vi "SFP_SwitchDMM.vi"(11 "DMM Instrument":refnum<class "DMM Instrument.lvclass">) -> ()   [LabVIEW 2025]
doc: "Copyright 2017 National Instruments Corporation\n\nLicensed under the Apache License, Version 2.0 (the \"License\"); you may not use this file except in compliance with the License. You may obtain a copy of the License at http://www.apache.org/licenses/LICENSE-2.0\nUnless required by applicable law or agreed to in writing, software distributed under the License is distributed on an \"AS IS\" BASIS, WITHOUT WARRANTIES OR CONDITIONS OF ANY KIND, either express or implied. See the License for the specific language governing permissions and limitations under the License."
uses:
  DMM Instrument.lvclass/DMM Instrument.ctl
  DMM Instrument.lvclass
  C:/Users/Public/Documents/Sandia National Labs/TSS Plugin/Abstract Engine.lvlibp/Plugin/Abstract/Abstract Instrument/Abstract Instrument.lvclass
  C:/Users/Public/Documents/Sandia National Labs/TSS Plugin/CEF.lvlibp/serializable node/CEF_serializable node.lvclass
  C:/Users/Public/Documents/Sandia National Labs/TSS Plugin/CEF.lvlibp/Node/CEF_Node.lvclass
  C:/Working copy/tss/Plugin/Engines/DMM/DMM Instrument/DMM Instrument.lvclass
  C:/Users/Public/Documents/Sandia National Labs/TSS Plugin/Interface.lvlibp/Analog Input/AI.lvclass
  C:/Users/Public/Documents/Sandia National Labs/TSS Plugin/Interface.lvlibp/Digital Input/DI.lvclass
  DMM configuration/DMM configuration.lvclass
  C:/Users/Public/Documents/Sandia National Labs/TSS Plugin/Abstract Engine.lvlibp/Plugin/Abstract/Instrument configuration/Instrument configuration.lvclass
  C:/Users/Public/Documents/Sandia National Labs/TSS Plugin/CEF.lvlibp/serializable configuration/CEF_serializable configuration.lvclass
  C:/Working copy/tss/Plugin/Engines/DMM/DMM configuration/DMM configuration.lvclass
panel:
  out "Channels":T1(array[cluster]) {"Measurement" format="%#_4p"}
  out "Instrument":string caption="Instrument ::"
  # "ch"
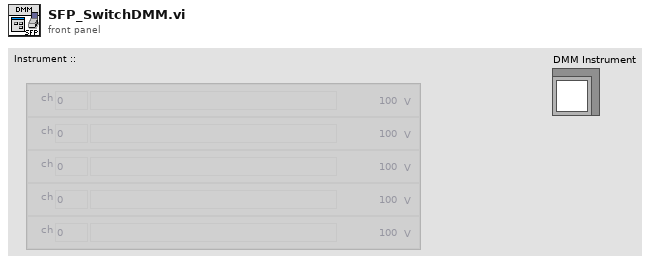
[diagram p1: front panel]
types:
  T1 = cluster{"Channel Alias":string, "Index":i32, "Measurement":dbl}[]
  T2 = enum32{"Invalid", "Default", "Floating", "Floating/Auto-Hide", "Modal"}
  T3 = typedef "Abstract Engine.lvlibp/Instrument configuration.lvclass/Default Instrument.ctl" = cluster{"Type":string, "Address":string, "SW Alias":string, "Description":string, "Enabled":bool}
  T4 = cluster{"Channel Alias":string, "Index":i32, "Measurement":dbl}
  T5 = typedef "Interface.lvlibp/AI.lvclass/Channel.ctl" = cluster{"Alias":string, "DataType":enum16{"Anaolg Input", "Waveform"}, "Unit":enum16{"---", "V", "A", "Ohm", "Hz", "uF", "degC", "deg"}, "Upper limit":dbl, "Lower limit":dbl, "Measurement":variant}
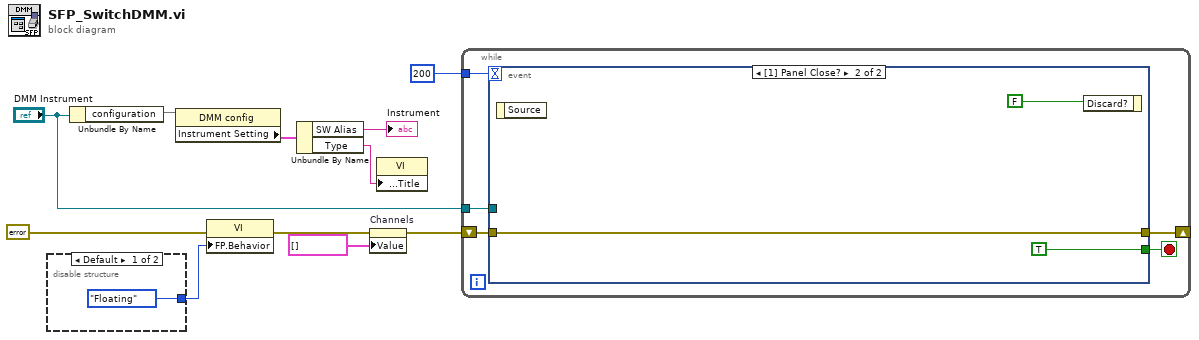
[diagram p0: block diagram]
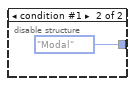
[diagram p2: hidden frame]
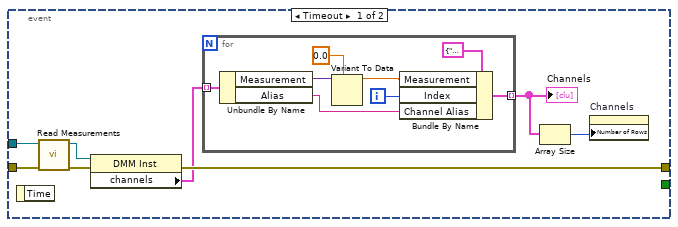
[diagram p3: hidden frame]
diagram:
  n1 = disable-structure shown="Default" {
    disable-tunnel: [T2."Floating" ("Front Panel Window:Behavior") T2."Modal" ("Front Panel Window:Behavior")] -> w9
    frame condition #0 (active) {
    }
    frame condition #1 {
    }
  }
  n2 = Unbundle By Name("DMM Instrument") -> ("configuration"=w7)
  n3 = property class="DMM config"(reference=w7) -> ("Instrument Setting"=w6:T3)  [unwired: 1 in, 2 out]
  n4 = property class="VI"(error in=errorcluster {"status"=FALSE, "code"=0, "source"=""} ("error in (no error)"), "FP.Behavior"=w9) -> (error out=w2:errorcluster)  [unwired: 1 in, 1 out]
  n5 = Unbundle By Name(w6) -> ("SW Alias"=→"Instrument":string, "Type"=w10:string)
  n6 = property on="Channels" class="Arr (strict)"(error in=w2, "Value"=T1 [] ("Channels")) -> (error out=w1:errorcluster)  [unwired: 1 in, 1 out]
  n7 = property class="VI"("Front Panel.Title"=w10) -> ()  [unwired: 2 in, 2 out]
  n8 = while {
    shift-right: [w16] -> _
    shift-left: w1 -> [w17]
    tunnel: 200 -> [w14]
    tunnel: "DMM Instrument" -> [w15]
    stop <- w18 stop-if-true
    n9 = event shown="[1] Panel Close?" {
      selector: _ -> [_ _]
      dyn-events: _ -> [_ _]
      timeout: w14 -> [_ _]
      tunnel: [_ TRUE] -> w18
      tunnel: [w21 w35] -> w16
      tunnel: w17 -> [w24 w35]
      tunnel: w15 -> [w26 _]
      event Timeout {
        n10 = event-data() -> ()  [unwired: 1 in, 1 out]
        n11 = call "Read Measurements.vi"("error in"=w24, "DMM Instrument"=w26) -> ("error out"=w23:errorcluster, "DMM Instrument out"=w20:refnum<class "DMM Instrument.lvclass">)  [unwired: 8 in]
        n12 = property class="DMM Inst"(reference=w20, error in=w23) -> (error out=w21:errorcluster, "channels"=w19:T5[])  [unwired: 1 out]
        n13 = for {
          tunnel: [w34] -> w22 mode=indexing
          tunnel: w19 -> [w32] mode=indexing
          i -> [w28]
          n14 = Unbundle By Name(w32) -> ("Measurement"=w31:variant, "Alias"=w27:string)
          n15 = Variant To Data(type=0.0 ("Measurement"), Variant=w31) -> (data=w29:dbl)  [unwired: 1 in, 1 out]
          n16 = Bundle By Name(cluster=T4 {"Channel Alias"="", "Index"=0, "Measurement"=0.0} ("Channel"), "Measurement"=w29, "Index"=w28, "Channel Alias"=w27) -> (w34:T4)
        }
        "Channels" <- w22
        n17 = Array Size(array=w22) -> (size(s)=w25:i32)
        n18 = property on="Channels" class="Arr (strict)"("Number of Rows"=w25) -> ()  [unwired: 2 in, 2 out]
      }
      event Panel Close? {
        n19 = event-data() -> ()  [unwired: 1 in, 1 out]
        n20 = event-data("Discard?"=FALSE) -> ()  [unwired: 1 in, 1 out]
      }
    }
  }
